vi "IND560 Decode Weight Data.vi"(8 "Error In":errorcluster, 11 "read buffer":string) -> (0 "Error Out":errorcluster, 2 "Displayed Net Wt.":dbl=0.04, 3 "Displayed Gross Wt.":dbl=2.91, 5 "Units":string)   [LabVIEW 2018]
panel:
  out "Array":string[](array[string])=["00C128~wt0101=        3.45^wt0102=        0.58", "00C130~wt0101=        3.42^wt0102=        0.55", "00C132~wt0101=        3.32^wt0102=        0.45", "00C134~wt0101=        3.22^wt0102=        0.35", "00C136~wt0101=        3.13^wt0102=        0.26", "00C138~wt0101=        3.03^wt0102=        0.16", "00C140~wt0101=        2.98^wt0102=        0.11", "00C142~wt0101=        2.94^wt0102=        0.07", "00C144~wt0101=        2.91^wt0102=        0.04"]
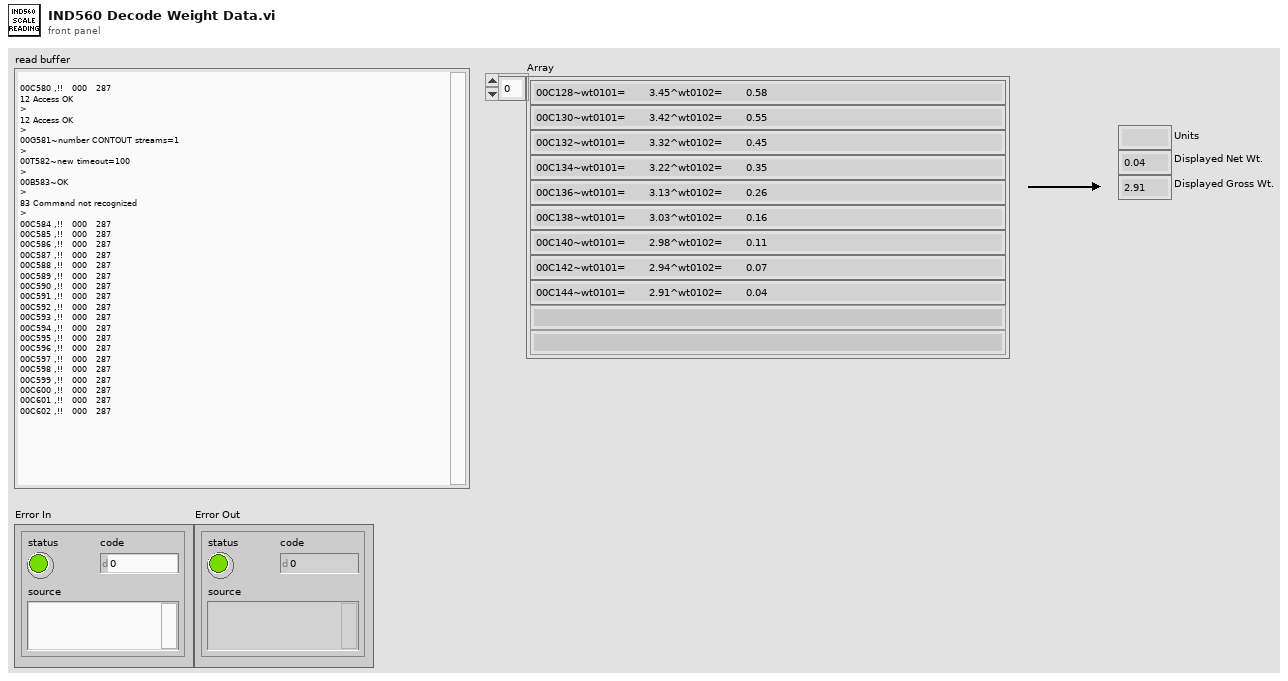
[diagram p1: front panel]
types:
  T1 = typedef "IND560 Data Output Selector.ctl" = enum16{"None", "Use Gross Not Equal Net", "Use Gross Equal Net", "Use Unstable Weights"}
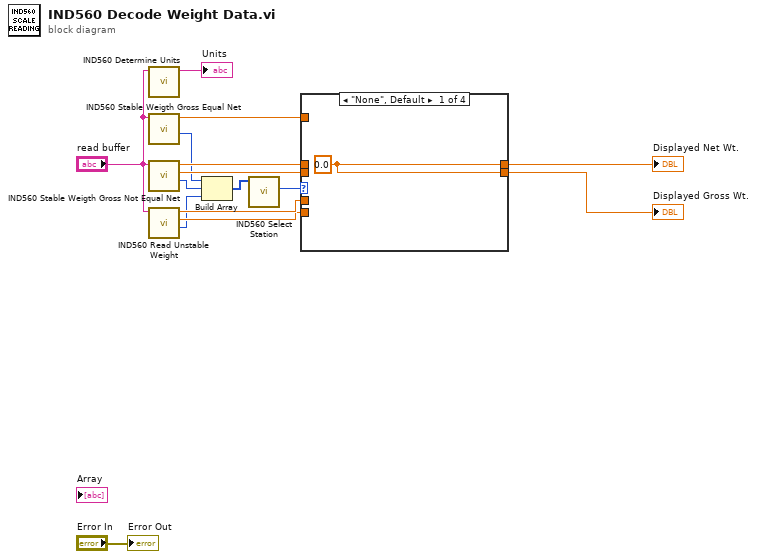
[diagram p0: block diagram]
diagram:
  n1 = call "IND560 Determine Units.vi"("read buffer"="read buffer") -> ("String"=→"Units":string)  [unwired: 9 in, 1 out]
  n2 = call "IND560 Stable Weigth Gross Equal Net.vi"("read buffer"="read buffer") -> ("IND560 Selector"=w5:T1, "Gross and Net Weight"=w11:dbl)  [unwired: 8 in, 1 out]
  n3 = call "IND560 Stable Weigth Gross Not Equal Net.vi"("read buffer"="read buffer") -> ("IND560 Selector"=w4:T1, "Gross Weight"=w6:dbl, "Net Weight"=w7:dbl)  [unwired: 7 in, 1 out]
  n4 = call "IND560 Read Unstable Weight.vi"("read buffer"="read buffer") -> ("IND560 Selector"=w3:T1, "Displayed Gross Wt."=w8:dbl, "Displayed Net Wt."=w9:dbl)  [unwired: 7 in, 1 out]
  n5 = Build Array(w5, w4, w3) -> (w2:T1[])
  n6 = call "IND560 Select Station.vi"("All Stations"=w2) -> ("IND560 Selector 2"=w1:T1)  [unwired: 10 in]
  n7 = case shown="\"None\", Default" w1 {
    tunnel: w8 -> [_ _ _ w20]
    tunnel: w9 -> [_ _ _ w21]
    tunnel: [w16 w17 w19 w20] -> w13
    tunnel: [w16 w18 w19 w21] -> w12
    tunnel: w11 -> [_ _ w19 _]
    tunnel: w7 -> [_ w18 _ _]
    tunnel: w6 -> [_ w17 _ _]
    frame "None", Default {
      w16 = 0.0 ("Displayed Net Wt.")
    }
    frame "Use Gross Not Equal Net" {
    }
    frame "Use Gross Equal Net" {
    }
    frame "Use Unstable Weights" {
    }
  }
  "Displayed Net Wt." <- w12
  "Displayed Gross Wt." <- w13
  "Error Out" <- "Error In"
